vi "Stream Arc On Axis Subset.vi"(0 "VISA resource name":refnum<visa-resource-name>, 1 "Center Point":i64[](array[numeric]), 2 "End Point":i64[](array[numeric]), 3 "Symbolic Axes":string[](array[string]), 5 "Stream Number (1)":u8=1, 9 "Device Number":string, 11 "error in (no error)":errorcluster, 12 "Position Mode (0: absolute)":u16(ring) items=["absolute", "relative"], 13 "Direction (0: clockwise)":u16(ring) items=["clockwise", "counter-clockwise"]) -> (4 "VISA resource name out":refnum<visa-resource-name>, 15 "error out":errorcluster)   [LabVIEW 2018, in "Zaber A Series.lvlib"]
doc: "Adds a circular arc command to an open stream using a subset of the stream's axes. The position where the previous stream command leaves the device will be the starting point for the arc. The Center Position input specifies where the center of the circle will be, and the End Point input specified the end of the arc. There is also a Direction input to control which way around the circle the arc is drawn.\n\nThe Position Mode input controls whether the center and endpoint positions are absolute or relative to the arc start.\n\nThe center and end points are specified in microstep units - use the Convert Position to Device Units VI to convert from standard measurements.\n\nThe Symbolic Axes input specifies which of the stream's axes the command will operate on. This should contain two letters as separate array entries. The entries in the Symbolic Axes input are not axis numbers but letters that map to axes in the order the axes were added to the stream. For example, if the stream was set up with axes [1, 3, 2] then the symbol definitions will be a = 1, b = 3, c = 2. You can also permute the order in this input, so if you pass Symbolic Axes the input [c, b] in this example, then the coordinates you give will be for physical axes [2, 3].\n\nArcs are only supported on two axes, so this VI should be used instead of the other Stream Arc VIs if your stream is set up with more than two axes.\n\nThis VI does not check in advance for error conditions such as streams not being supported or the stream not being open.\n\nThis VI requires that the device have Firmware version 7, that the Initialize VI has been called with the same serial port and that the specified stream is open."
uses:
  Zaber A Series.lvlib
  Private/All Commands.ctl
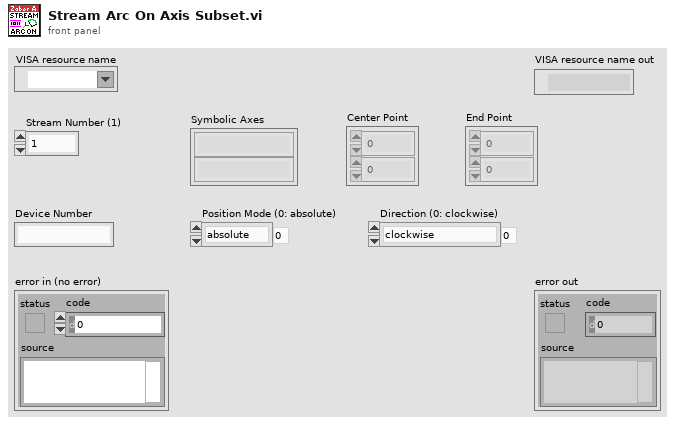
[diagram p1: front panel]
types:
  T1 = typedef "Zaber A Series.lvlib/All Commands.ctl" = string
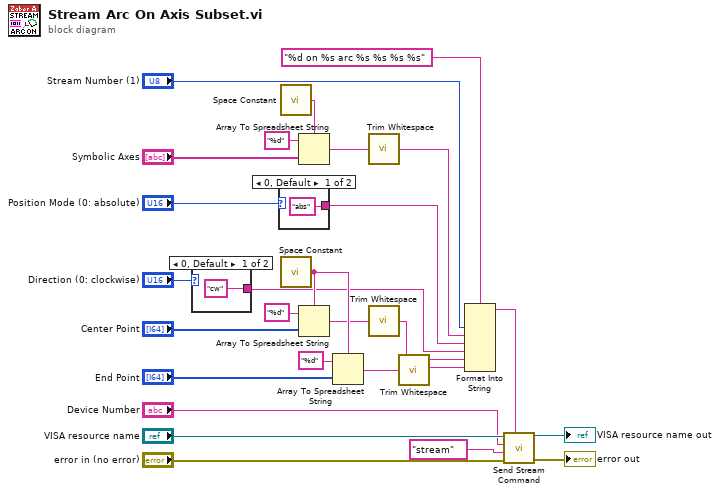
[diagram p0: block diagram]
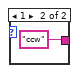
[diagram p2: hidden frame]
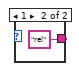
[diagram p3: hidden frame]
diagram:
  n1 = case shown="0, Default" "Direction (0: clockwise)" {
    tunnel: ["cw" "ccw"] -> w7
    frame 0, Default {
    }
    frame 1 {
    }
  }
  n2 = case shown="0, Default" "Position Mode (0: absolute)" {
    tunnel: ["abs" "rel"] -> w6
    frame 0, Default {
    }
    frame 1 {
    }
  }
  n3 = call <vilib>:"Space Constant.vi"() -> ("String"=w4:string)
  n4 = call <vilib>:"Space Constant.vi"() -> ("String"=w17:string)
  n5 = Array To Spreadsheet String(delimiter (Tab)=w4, array="Symbolic Axes", 3:"%d" ("format string")) -> (spreadsheet string=w5:string)
  n6 = Array To Spreadsheet String(delimiter (Tab)=w17, array="Center Point", 3:"%d" ("format string")) -> (spreadsheet string=w16:string)
  n7 = Array To Spreadsheet String(delimiter (Tab)=w17, array="End Point", 3:"%d" ("format string")) -> (spreadsheet string=w15:string)
  n8 = call <vilib>:"Trim Whitespace.vi"("string"=w5) -> ("trimmed string"=w2:string)  [unwired: 1 in]
  n9 = call <vilib>:"Trim Whitespace.vi"("string"=w16) -> ("trimmed string"=w8:string)  [unwired: 1 in]
  n10 = call <vilib>:"Trim Whitespace.vi"("string"=w15) -> ("trimmed string"=w9:string)  [unwired: 1 in]
  n11 = Format Into String(format string="%d on %s arc %s %s %s %s", "Stream Number (1)", w2, w6, w7, w8, w9) -> (resulting string=w12:string)  [unwired: 2 in, 1 out]
  n12 = call "Send Stream Command.vi"("Data"=w12, "error in (no error)"="error in (no error)", "Command"=T1 "stream" ("Complete Command List"), "Device Number"="Device Number", "VISA resource name"="VISA resource name") -> ("error out"=→"error out":errorcluster, "VISA resource name out"=→"VISA resource name out":refnum<visa-resource-name>)  [unwired: 5 in]
